vi "LVPortCallMatlabUpdate.vi"(10 "pID":string, 11 "Value Type (Or value to update)":variant) -> ()   [LabVIEW 2017]
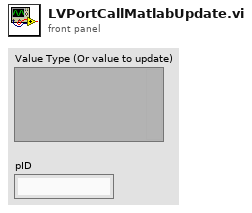
[diagram p1: front panel]
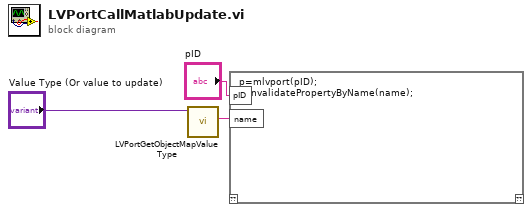
[diagram p0: block diagram]
diagram:
  n1 = call "LVPortGetObjectMapValueType.vi"("Value"="Value Type (Or value to update)") -> ("Name"=w3:string)  [unwired: 6 in, 4 out]
  n2 = script code="p=mlvport(pID);\np.InvalidatePropertyByName(name);"("pID"="pID", "name"=w3) -> ()  [unwired: 1 in, 1 out]
